vi "Teleop.vi"(10 "Match Info":T1={"Autonomous Elapsed Seconds"=0.0, "TeleOp Elapsed Seconds"=0.0, "Disabled Elapsed Seconds"=0.0, "Visited Autonomous"=FALSE, "Visited TeleOp"=FALSE, "Visited Disabled"=FALSE, "Autonomous Settings"={"Autonomous Style"=enum."Independent", "VI Refnum"=refnum}}, 11 "Call Context":T2) -> ()   [LabVIEW 2016]
doc: "This VI is called for each TeleOp packet received from the DS where the robot is not disabled. It is often used to read from the joysticks and update I/O or to update setpoints for timed control loops. It should complete and return within 20 milliseconds or it may miss DS packets."
uses:
  <vilib>/Rock Robotics/WPI/DriverStation/WPI_DriverStationDerivedRobotMode.ctl
  <vilib>/Rock Robotics/WPI/DriverStation/WPI_DriverStationMatch Info.ctl
  jystickModes.ctl
  <vilib>/Rock Robotics/Network Tables/NT Read Boolean.vi
  <vilib>/Rock Robotics/Network Tables/NT Read Number.vi
  <vilib>/Rock Robotics/WPI/Utilities/WPI_GetSetVariantRefNum.vi
  <vilib>/Rock Robotics/Network Tables/NT Write Boolean Array.vi
  <vilib>/Rock Robotics/Network Tables/NT Write Numeric Array.vi
panel:
  out "Sample Slider 0":dbl(slide) scale=0.0..5.0
  out "Sample Boolean 1":bool
  out "Sample Boolean 0":bool
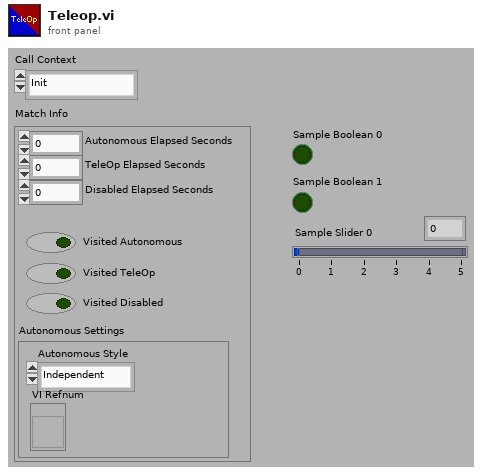
[diagram p1: front panel]
types:
  T1 = typedef "WPI_DriverStationMatch Info.ctl" = cluster{"Autonomous Elapsed Seconds":dbl, "TeleOp Elapsed Seconds":dbl, "Disabled Elapsed Seconds":dbl, "Visited Autonomous":bool, "Visited TeleOp":bool, "Visited Disabled":bool, "Autonomous Settings":cluster{"Autonomous Style":enum16{"Iterative", "Independent"}, "VI Refnum":refnum<vi>}}
  T2 = typedef "WPI_DriverStationDerivedRobotMode.ctl" = enum16{"Init", "Execute", "Stop"}
  T3 = typedef "jystickModes.ctl" = enum16{"Arcade Joystick", "Tank", "Xbox top", "Xbox Right"}
  T4 = typedef "WPI_RobotDriveDevRef.ctl" = cluster{"DevStatus":errorcluster, "Motors[]":T5[], "Square Inputs":bool, "Max Output":dbl}
  T5 = typedef "WPI_MotorControlDeviceRef.ctl" = cluster{"DeviceStatus":errorcluster, "Type":T6, "PWM":cluster{"PWM Channel":T7, "DeadBand":T8}, "CAN":cluster{"Device Number":u8, "SetOutput VI Ref":variant, "GetOutput VI Ref":variant, "Enable VI Ref":variant, "Disable VI Ref":variant, "Data":variant}, "Invert":bool}
  T6 = typedef "WPI_MotorControlType.ctl" = enum16{"PWM", "CAN"}
  T7 = typedef "FPGA_DIOPWMChannel.ctl" = enum8{"PWM 0", "PWM 1", "PWM 2", "PWM 3", "PWM 4", "PWM 5", "PWM 6", "PWM 7", "PWM 8", "PWM 9", "PWM MXP 0", "PWM MXP 1", "PWM MXP 2", "PWM MXP 3", "PWM MXP 4", "PWM MXP 5", "PWM MXP 6", "PWM MXP 7", "PWM MXP 8", "PWM MXP 9", "Invalid"}
  T8 = typedef "WPI_PWMDeadband.ctl" = cluster{"Name":string, "maxPositivePwm":i32, "minPositivePwm":i32, "centerPwm":i32, "maxNegativePwm":i32, "minNegativePwm":i32, "angularRange":u16}
  T9 = typedef "WPI_JoystickDevRef.ctl" = cluster{"Device":T10}
  T10 = typedef "WPI_JoystickDeviceEnum.ctl" = enum16{"USB 0", "USB 1", "USB 2", "USB 3", "USB 4", "USB 5"}
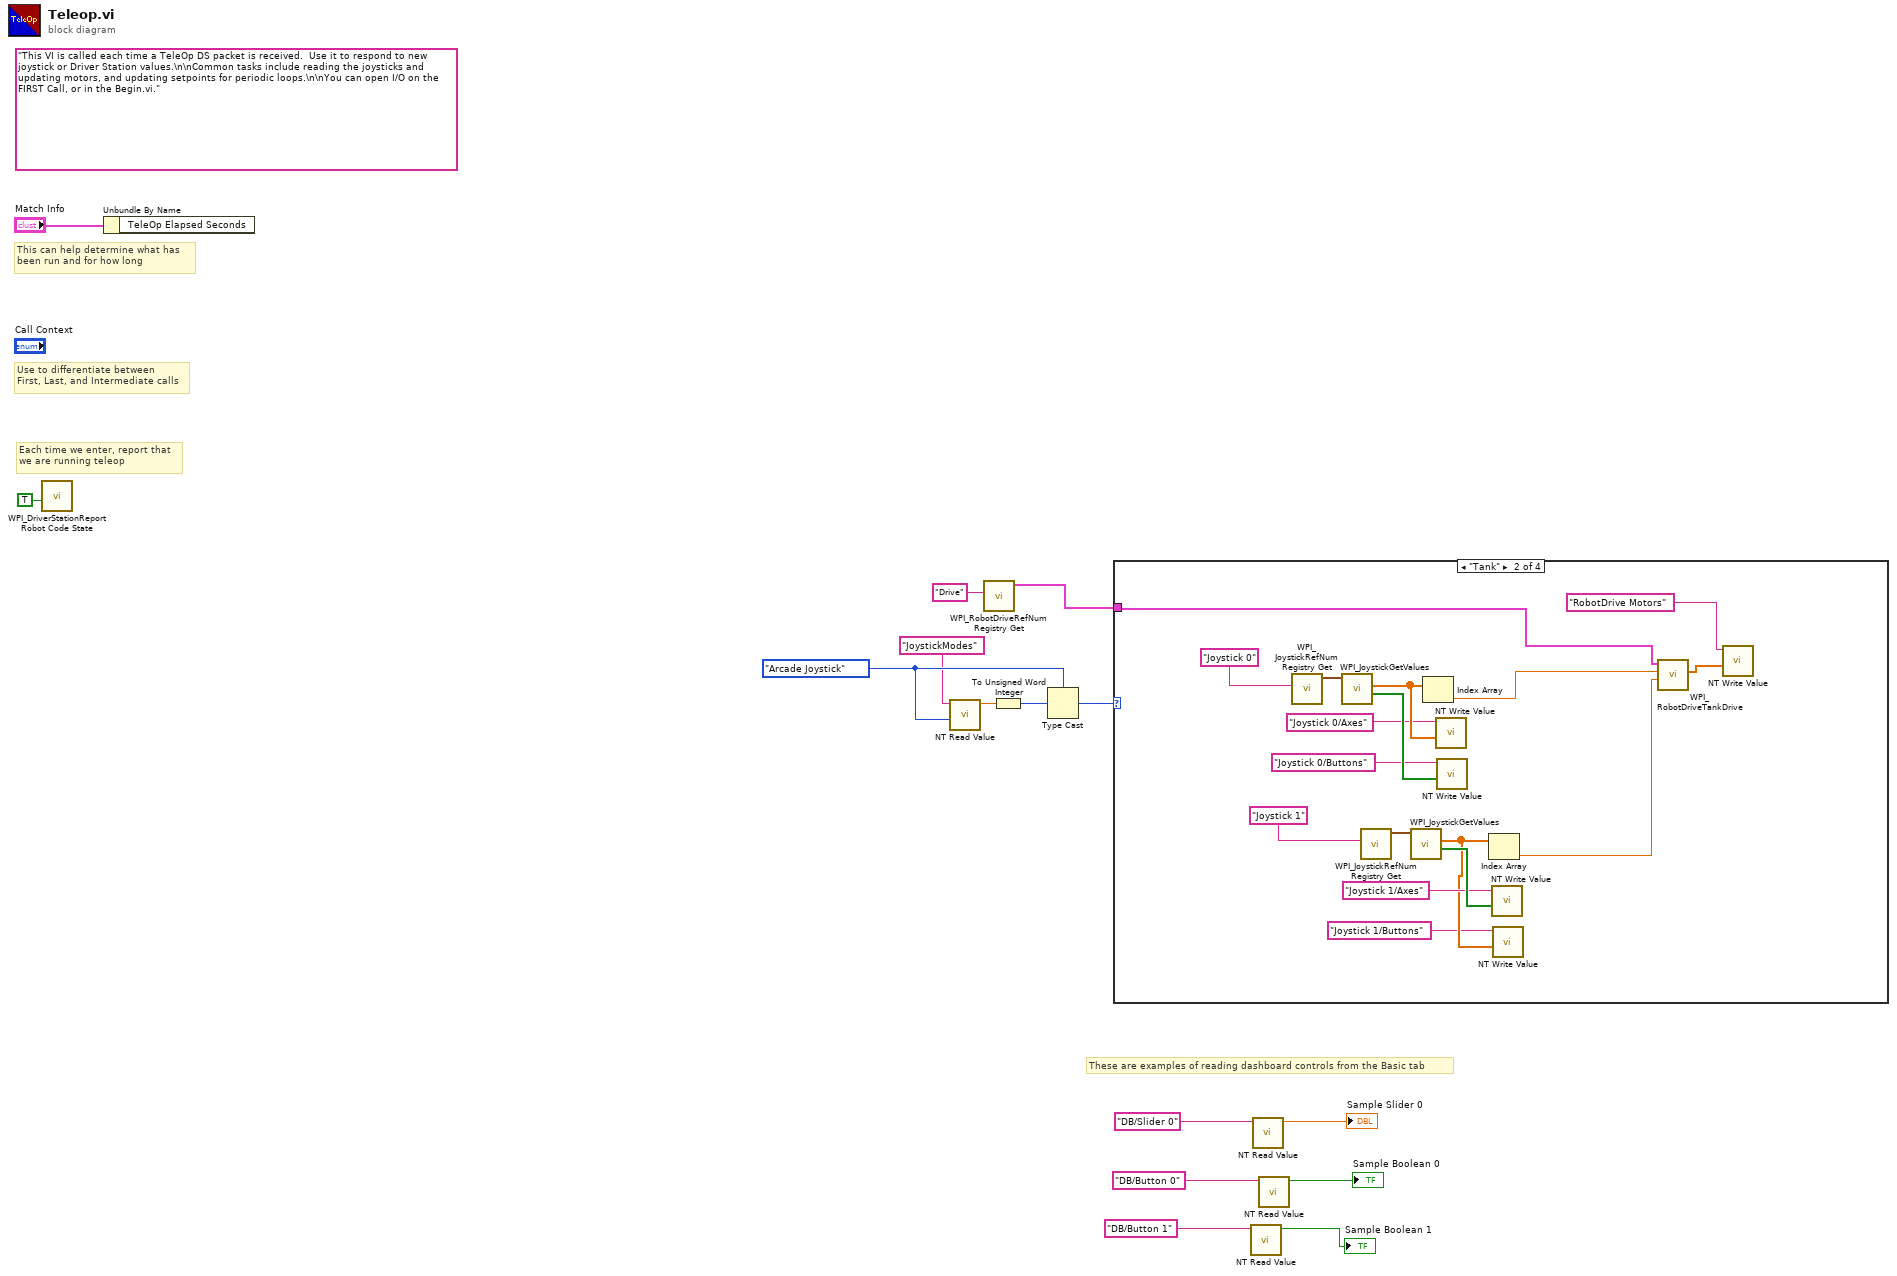
[diagram p0: block diagram]
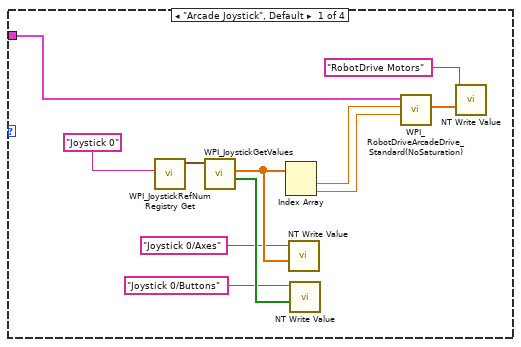
[diagram p2: hidden frame]
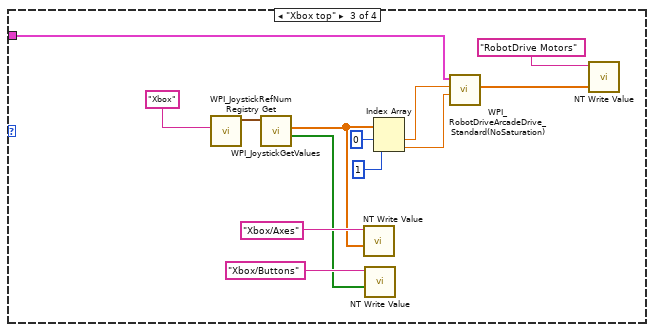
[diagram p3: hidden frame]
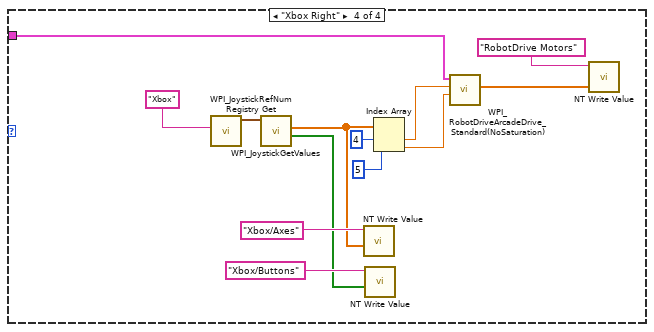
[diagram p4: hidden frame]
diagram:
  w3 = jystickModes."Arcade Joystick"
  (unwired) "This VI is called each time a TeleOp DS packet is received.  Use it to respond to new joystick or Driver Station values.\n\nCommon tasks include reading the joysticks and updating motors, and updating setpoints for periodic loops.\n\nYou can open I/O on the FIRST Call, or in the Begin.vi."
  # "These are examples of reading dashboard controls from the Basic tab"
  # "Each time we enter, report that\nwe are running teleop"
  # "Use to differentiate between\nFirst, Last, and Intermediate calls"
  # "This can help determine what has\nbeen run and for how long"
  n1 = call <vilib>:"WPI_DriverStationReport Robot Code State.vi"("TeleOp"=TRUE ("Autonomous")) -> ()  [unwired: 10 in, 1 out]
  n2 = Unbundle By Name("Match Info") -> ()  [unwired: 1 out]
  n3 = call-poly <vilib>:"NT Read Value.vi"("Default Value"=w3, "Name"="JoystickModes") -> ("Numeric"=w5:dbl)  [unwired: 8 in, 1 out]
  n4 = call <vilib>:"WPI_RobotDriveRefNum Registry Get.vi"("refnum name"="Drive") -> ("RobotDriveDevRef"=w7:T4)  [unwired: 1 in, 9 out]
  n5 = To Unsigned Word Integer(number=w5) -> (unsigned 16bit integer=w2:u16)
  n6 = Type Cast(type=w3, x=w2) -> (*(type *) &x=w4:T3)
  n7 = case shown="\"Tank\"" w4 {
    tunnel: w7 -> [w18 w28 w47 w60]
    frame "Arcade Joystick", Default {
      n8 = call <vilib>:"WPI_JoystickRefNum Registry Get.vi"("refnum name"="Joystick 0") -> ("JoystickDevRef"=w22:T9)  [unwired: 1 in, 9 out]
      n9 = call <vilib>:"WPI_JoystickGetValues.vi"("JoystickDevRef"=w22) -> ("Buttons"=w26:bool[], "Axes"=w25:dbl[])  [unwired: 6 in, 3 out]
      n10 = Index Array(array=w25) -> (element #1=w20:dbl, element #2=w23:dbl)  [unwired: 2 in]
      n11 = call-poly <vilib>:"NT Write Value.vi"("Numeric Array"=w25, "Name"="Joystick 0/Axes") -> ()  [unwired: 9 in, 1 out]
      n12 = call-poly <vilib>:"NT Write Value.vi"("Boolean Array"=w26, "Name"="Joystick 0/Buttons") -> ()  [unwired: 9 in, 1 out]
      n13 = call <vilib>:"WPI_RobotDriveArcadeDrive_Standard(NoSaturation).vi"("Y axis value"=w23, "X axis value"=w20, "RobotDriveDevRef"=w18) -> ("Motor Values"=w19:dbl[])  [unwired: 1 in, 7 out]
      n14 = call-poly <vilib>:"NT Write Value.vi"("Numeric Array"=w19, "Name"="RobotDrive Motors") -> ()  [unwired: 9 in, 1 out]
    }
    frame "Tank" {
      n15 = call <vilib>:"WPI_JoystickRefNum Registry Get.vi"("refnum name"="Joystick 0") -> ("JoystickDevRef"=w30:T9)  [unwired: 1 in, 9 out]
      n16 = call <vilib>:"WPI_JoystickGetValues.vi"("JoystickDevRef"=w30) -> ("Buttons"=w33:bool[], "Axes"=w36:dbl[])  [unwired: 6 in, 3 out]
      n17 = call <vilib>:"WPI_JoystickRefNum Registry Get.vi"("refnum name"="Joystick 1") -> ("JoystickDevRef"=w35:T9)  [unwired: 1 in, 9 out]
      n18 = call <vilib>:"WPI_JoystickGetValues.vi"("JoystickDevRef"=w35) -> ("Buttons"=w40:bool[], "Axes"=w38:dbl[])  [unwired: 6 in, 3 out]
      n19 = Index Array(array=w36) -> (element=w41:dbl)  [unwired: 1 in]
      n20 = call-poly <vilib>:"NT Write Value.vi"("Numeric Array"=w36, "Name"="Joystick 0/Axes") -> ()  [unwired: 9 in, 1 out]
      n21 = call-poly <vilib>:"NT Write Value.vi"("Boolean Array"=w33, "Name"="Joystick 0/Buttons") -> ()  [unwired: 9 in, 1 out]
      n22 = Index Array(array=w38) -> (element=w42:dbl)  [unwired: 1 in]
      n23 = call-poly <vilib>:"NT Write Value.vi"("Boolean Array"=w40, "Name"="Joystick 1/Axes") -> ()  [unwired: 9 in, 1 out]
      n24 = call-poly <vilib>:"NT Write Value.vi"("Numeric Array"=w38, "Name"="Joystick 1/Buttons") -> ()  [unwired: 9 in, 1 out]
      n25 = call <vilib>:"WPI_RobotDriveTankDrive.vi"("Right axis value"=w42, "Left axis value"=w41, "RobotDriveDevRef"=w28) -> ("Motor Values"=w43:dbl[])  [unwired: 6 in, 2 out]
      n26 = call-poly <vilib>:"NT Write Value.vi"("Numeric Array"=w43, "Name"="RobotDrive Motors") -> ()  [unwired: 9 in, 1 out]
    }
    frame "Xbox top" {
      n27 = call <vilib>:"WPI_JoystickRefNum Registry Get.vi"("refnum name"="Xbox") -> ("JoystickDevRef"=w56:T9)  [unwired: 1 in, 9 out]
      n28 = call <vilib>:"WPI_JoystickGetValues.vi"("JoystickDevRef"=w56) -> ("Buttons"=w52:bool[], "Axes"=w51:dbl[])  [unwired: 6 in, 3 out]
      n29 = call-poly <vilib>:"NT Write Value.vi"("Numeric Array"=w51, "Name"="Xbox/Axes") -> ()  [unwired: 9 in, 1 out]
      n30 = call-poly <vilib>:"NT Write Value.vi"("Boolean Array"=w52, "Name"="Xbox/Buttons") -> ()  [unwired: 9 in, 1 out]
      n31 = Index Array(array=w51, index #1=0 ("index"), index #2=1 ("index")) -> (element #1=w49:dbl, element #2=w48:dbl)
      n32 = call <vilib>:"WPI_RobotDriveArcadeDrive_Standard(NoSaturation).vi"("Y axis value"=w48, "X axis value"=w49, "RobotDriveDevRef"=w47) -> ("Motor Values"=w50:dbl[])  [unwired: 1 in, 7 out]
      n33 = call-poly <vilib>:"NT Write Value.vi"("Numeric Array"=w50, "Name"="RobotDrive Motors") -> ()  [unwired: 9 in, 1 out]
    }
    frame "Xbox Right" {
      n34 = call <vilib>:"WPI_JoystickRefNum Registry Get.vi"("refnum name"="Xbox") -> ("JoystickDevRef"=w69:T9)  [unwired: 1 in, 9 out]
      n35 = call <vilib>:"WPI_JoystickGetValues.vi"("JoystickDevRef"=w69) -> ("Buttons"=w65:bool[], "Axes"=w64:dbl[])  [unwired: 6 in, 3 out]
      n36 = call-poly <vilib>:"NT Write Value.vi"("Numeric Array"=w64, "Name"="Xbox/Axes") -> ()  [unwired: 9 in, 1 out]
      n37 = call-poly <vilib>:"NT Write Value.vi"("Boolean Array"=w65, "Name"="Xbox/Buttons") -> ()  [unwired: 9 in, 1 out]
      n38 = Index Array(array=w64, index #1=4 ("index"), index #2=5 ("index")) -> (element #1=w62:dbl, element #2=w61:dbl)
      n39 = call <vilib>:"WPI_RobotDriveArcadeDrive_Standard(NoSaturation).vi"("Y axis value"=w61, "X axis value"=w62, "RobotDriveDevRef"=w60) -> ("Motor Values"=w63:dbl[])  [unwired: 1 in, 7 out]
      n40 = call-poly <vilib>:"NT Write Value.vi"("Numeric Array"=w63, "Name"="RobotDrive Motors") -> ()  [unwired: 9 in, 1 out]
    }
  }
  n41 = call-poly <vilib>:"NT Read Value.vi"("Name"="DB/Button 1" ("refnum name")) -> ("Boolean"=→"Sample Boolean 1":bool)  [unwired: 9 in, 1 out]
  n42 = call-poly <vilib>:"NT Read Value.vi"("Name"="DB/Slider 0" ("refnum name")) -> ("Numeric"=→"Sample Slider 0":dbl)  [unwired: 9 in, 1 out]
  n43 = call-poly <vilib>:"NT Read Value.vi"("Name"="DB/Button 0" ("refnum name")) -> ("Boolean"=→"Sample Boolean 0":bool)  [unwired: 9 in, 1 out]
